vi "Extract Payload_length (SubVI).vi"(11 "data in":string) -> (1 "Residus_length":u32, 2 "Payload_length":u32, 3 "Total_Length":i32)   [LabVIEW 2015]
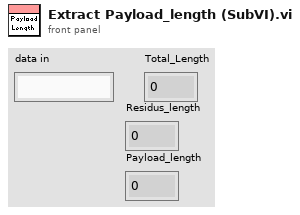
[diagram p1: front panel]
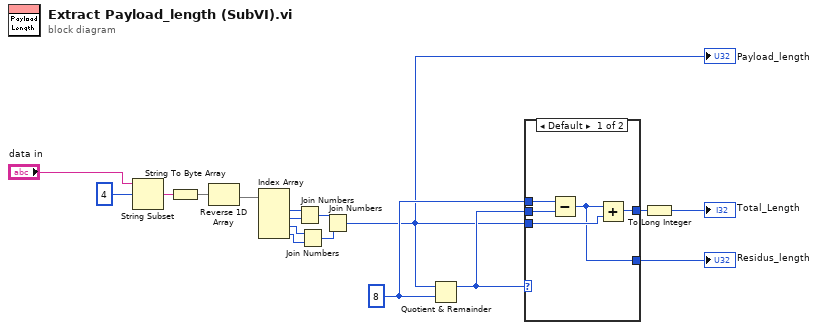
[diagram p0: block diagram]
diagram:
  w15 = u32 8 ("y")
  n1 = String Subset(string="data in", offset (0)=4) -> (substring=w5:string)  [unwired: 1 in]
  n2 = String To Byte Array(string=w5) -> (unsigned byte array=w6:u8[])
  n3 = Reverse 1D Array(array=w6) -> (reversed array=w7:u8[])
  n4 = Index Array(array=w7) -> (element #1=w8:u8, element #2=w9:u8, element #3=w10:u8, element #4=w11:u8)  [unwired: 4 in]
  n5 = Join Numbers(hi=w8, lo=w9) -> ((hi.lo)=w12:u16)
  n6 = Join Numbers(hi=w10, lo=w11) -> ((hi.lo)=w13:u16)
  n7 = Join Numbers(hi=w12, lo=w13) -> ((hi.lo)=w14:u32)
  "Payload_length" <- w14
  n8 = Quotient & Remainder(x=w14, y=w15) -> (x-y*floor(x/y)=w16:u32)  [unwired: 1 out]
  n9 = case shown="Default" w16 {
    tunnel: w14 -> [w20 w23]
    tunnel: [w19 w23] -> w17
    tunnel: w15 -> [w22 _]
    tunnel: w16 -> [w21 _]
    tunnel: [w18 _] -> w2
    frame Default {
      n10 = Subtract(x=w22, y=w21) -> (x-y=w18:u32)
      n11 = Add(x=w18, y=w20) -> (x+y=w19:u32)
    }
    frame 0 {
    }
  }
  "Residus_length" <- w2
  n12 = To Long Integer(number=w17) -> (32bit integer=→"Total_Length":i32)
